vi "DataLog Read Last String.vi"(7 "tag":string, 9 "tag index in (name lookup)":i32=-1, 11 "error in (no error)":errorcluster) -> (4 "string":string, 6 "time":dbl format="%<%H:%M:%S%2u\n%Y/%m/%d>T", 10 "tag index out":i32, 15 "error out":errorcluster)   [LabVIEW 2012]
doc: "Reads the last-written string (the current value) from a string tag of the live database."
uses:
  typedefs/t_DataLog Live Tag Strings Methods.ctl
  typedefs/t_DataLog Tag Hash Methods.ctl
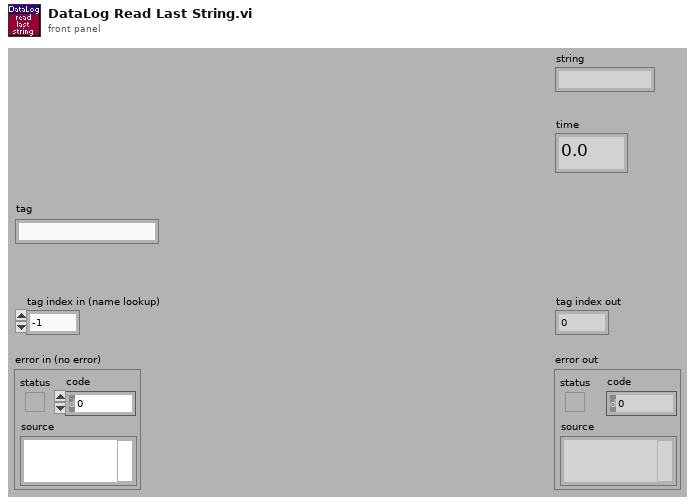
[diagram p1: front panel]
types:
  T1 = typedef "t_DataLog Live Tag Strings Methods.ctl" = enum16{"initialize", "rebuffer", "read", "write", "cleanup"}
  T2 = typedef "t_DataLog Tag Hash Methods.ctl" = enum16{"initialize", "add tag", "index tag", "lookup", "#tags", "cleanup", "write recovery", "read recovery", "delete recovery"}
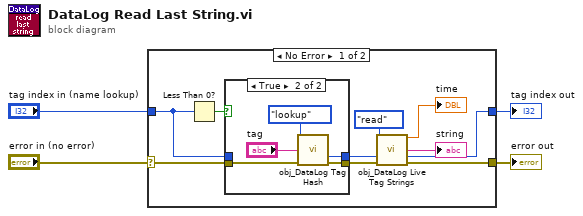
[diagram p0: block diagram]
diagram:
  n1 = case shown="No Error" "error in (no error)" {
    selector: "error in (no error)" -> [w11 w23]
    tunnel: [w5 w23] -> w3
    tunnel: "tag index in (name lookup)" -> [w10 w22]
    tunnel: [w7 w22] -> w1
    frame No Error {
      n2 = Less Than 0?(x=w10) -> (x < 0?=w12:bool)
      n3 = case shown="True" w12 {
        tunnel: w11 -> [w16 w21]
        tunnel: [w16 w19] -> w9
        tunnel: [w15 w18] -> w6
        tunnel: w10 -> [w15 _]
        frame False {
        }
        frame True {
          n4 = call "obj_DataLog Tag Hash.vi"("method"=t_DataLog_Tag_Hash_Methods."lookup", "tag in"="tag", "error in (no error)"=w21) -> ("tag index out"=w18:i32, "error out"=w19:errorcluster)  [unwired: 9 in, 2 out]
        }
      }
      n5 = call "obj_DataLog Live Tag Strings.vi"("method"=t_DataLog_Live_Tag_Strings_Methods."read", "tag index"=w6, "error in (no error)"=w9) -> ("time"=→"time":dbl, "string out"=→"string":string, "dup tag index"=w7:i32, "error out"=w5:errorcluster)  [unwired: 9 in]
    }
    frame Error {
    }
  }
  "error out" <- w3
  "tag index out" <- w1
